vi "Initialize.vi"(8 "error in (no error)":errorcluster) -> (0 "error out":errorcluster, 1 "update interval":dbl=10.0, 3 "config":T1)   [LabVIEW 2017, in "DeviceHealth.lvlib"]
uses:
  <vilib>/addons/InsightCM/Devices/Shared/Common/DeviceHealth/DeviceHealth.lvlib
  <vilib>/addons/InsightCM/Devices/Shared/Common/DeviceHealth/controls/config.ctl
  <vilib>/addons/InsightCM/Devices/Shared/Common/DeviceHealth/controls/deviceHealthTag.ctl
  <vilib>/addons/InsightCM/Devices/Shared/Common/DeviceHealth/controls/SystemHealthTagEnum.ctl
  <vilib>/addons/InsightCM/MessageBus/Base/controls/Tag.ctl
  <vilib>/addons/InsightCM/MessageBus/Base/controls/KeyValuePair.ctl
  <vilib>/addons/InsightCM/Utilities/PropertyHelpers/PropertyHelpers.lvlib
  <vilib>/addons/InsightCM/Utilities/GlobalConfiguration/GlobalConfiguration.lvlib
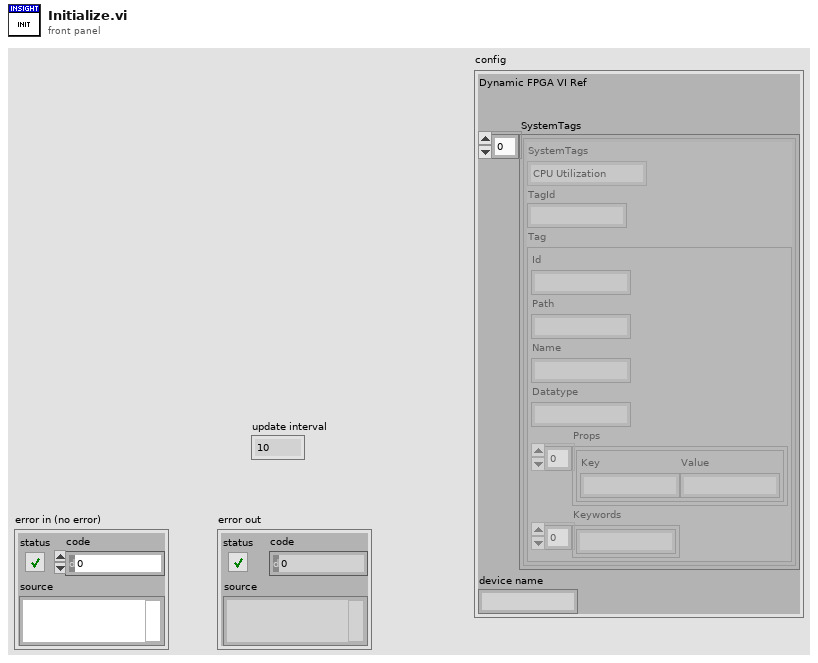
[diagram p1: front panel]
types:
  T1 = typedef "DeviceHealth.lvlib/config.ctl" = cluster{"Dynamic FPGA VI Ref":refnum<k20>, "SystemTags":T2[], "device name":string}
  T2 = typedef "DeviceHealth.lvlib/deviceHealthTag.ctl" = cluster{"SystemTags":T3, "TagId":string, "Tag":T4}
  T3 = typedef "DeviceHealth.lvlib/SystemHealthTagEnum.ctl" = enum16{"CPU Utilization", "Memory Utilization", "Disk Utilization", "Total Physical Memory", "Primary Disk Free", "Chassis Temperature", "LowRateCount"}
  T4 = typedef "Tag.ctl" = cluster{"Id":string, "Path":string, "Name":string, "Datatype":string, "Props":T5[], "Keywords":string[]}
  T5 = typedef "KeyValuePair.ctl" = cluster{"Key":string, "Value":string}
  T6 = typedef "SectionKeyValues.ctl" = cluster{"Section":string, "KeyValues":T5[]}
  T7 = typedef "R2_Device.ctl" = cluster{"Id":string, "Name":string, "DeviceType":string, "HardwareName":string, "IpAddress":string, "HardwareInfo":T5[], "ApplicationType":string, "ApplicationVersion":string, "EquipmentIds":string[], "ConfigurationVersion":string, "State":T8, "Properties":T5[], "DataGroups":T9[], "BurstModeTrigger":T13}
  T8 = typedef "DeviceState.ctl" = cluster{"Disabled":bool}
  T9 = typedef "R2_DataGroup.ctl" = cluster{"Name":string, "OperatingStates":T10[], "Properties":T5[], "EquipmentIds":string[], "AssetNodeId":string}
  T10 = typedef "OperatingState.ctl" = cluster{"Name":string, "Properties":T5[], "Triggers":T11[]}
  T11 = typedef "Trigger.ctl" = cluster{"Type":string, "Expression":string, "Conditions":T12[]}
  T12 = typedef "Condition.ctl" = cluster{"Source":string, "Type":string, "Operator":string, "CompareTo":string, "DwellSeconds":dbl}
  T13 = typedef "BurstModeTrigger.ctl" = cluster{"Trigger":T11, "SampleRate":string, "AcquisitionLength":string}
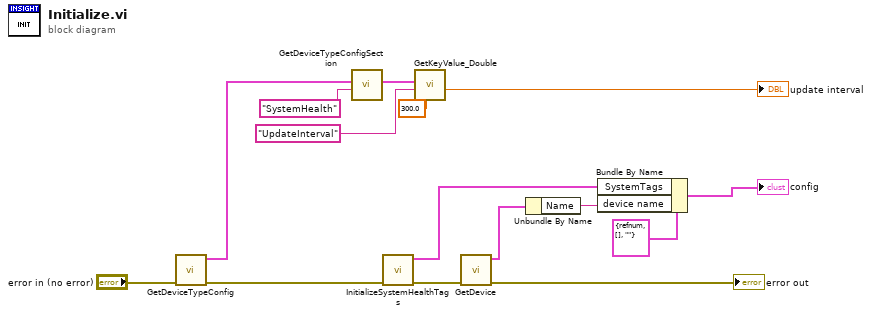
[diagram p0: block diagram]
diagram:
  n1 = call <vilib>:"GetDeviceTypeConfig.vi"("error in (no error)"="error in (no error)") -> ("error out"=w8:errorcluster, "key values"=w11:T6[])  [unwired: 8 in, 1 out]
  n2 = call <vilib>:"GetDeviceTypeConfigSection.vi"("key"="SystemHealth", "key values"=w11) -> ("key value pairs out"=w2:T5[])  [unwired: 8 in, 1 out]
  n3 = call <vilib>:"InitializeSystemHealthTags.vi"("error in (no error)"=w8) -> ("error out"=w6:errorcluster, "health tags"=w15:T2[])  [unwired: 9 in]
  n4 = call <vilib>:"GetKeyValue_Double.vi"("default"=300.0, "key"="UpdateInterval", "key value pairs"=w2) -> ("value"=→"update interval":dbl)  [unwired: 6 in, 2 out]
  n5 = call <vilib>:"GetDevice.vi"("error in (no error)"=w6) -> ("error out"=→"error out":errorcluster, "device configuration"=w5:T7)  [unwired: 8 in, 1 out]
  n6 = Unbundle By Name(w5) -> ("Name"=w4:string)
  n7 = Bundle By Name(cluster=T1 {"Dynamic FPGA VI Ref"=refnum, "SystemTags"=[], "device name"=""} ("config"), "SystemTags"=w15, "device name"=w4) -> (→"config":T1)
